vi "AV Write Array.vi"(8 "error in":errorcluster, 10 "Humidity AV":dbl[](array[numeric]), 11 "Humidity Actual Value in":refnum<class "Humidity Actual Value.lvclass">) -> (0 "error out":errorcluster, 3 "Humidity Actual Value out":refnum<class "Humidity Actual Value.lvclass">)   [LabVIEW 2023, in "Humidity Actual Value.lvclass"]
uses:
  Humidity Actual Value.lvclass
  Parents/Actual Value/Actual Value.lvclass
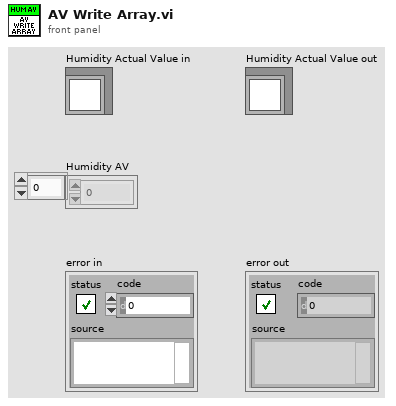
[diagram p1: front panel]
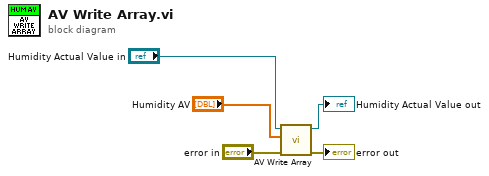
[diagram p0: block diagram]
diagram:
  n1 = call-parent "AV Write Array.vi"("error in"="error in", "Actual Value"="Humidity AV", "Actual Value in"="Humidity Actual Value in") -> ("error out"=→"error out":errorcluster, "Actual Value out"=→"Humidity Actual Value out":refnum<class "Humidity Actual Value.lvclass">)  [unwired: 7 in]
